vi "Tx1_Rx2_Acquisition.vi"(0 "DAQmx Device Name":tag, 1 "Tx Sampling Rate":dbl, 2 "Transmit Duration":dbl, 3 "Tx Amplitude":dbl=1.0 format="%0.2p", 5 "Tx Waveform":waveform(dbl)={"t0"=timestamp(0 s since 1904-01-01), "dt"=0.0, "Y"=[]}, 7 "AO Trigger Source":tag, 11 "error in":errorcluster, 12 "Rx Sampling Rate":dbl, 13 "Receive Duration":dbl, 14 "Voltage Rails":dbl) -> (4 "Rx Data":waveform(dbl)[](array[waveform]), 6 "Tx Waveform":waveform(dbl)(graph), 15 "error out":errorcluster)   [LabVIEW 2023]
uses:
  <vilib>/DAQmx/write.llb/DAQmx Write (Analog Wfm 1Chan NSamp).vi
  <vilib>/DAQmx/read.llb/DAQmx Read (Analog 1D Wfm NChan NSamp).vi
  <vilib>/DAQmx/create/channels.llb/DAQmx Create Channel (AO-Voltage-Basic).vi
  <vilib>/DAQmx/configure/timing.llb/DAQmx Timing (Sample Clock).vi
  <vilib>/DAQmx/configure/trigger.llb/DAQmx Start Trigger (Digital Edge).vi
  <vilib>/DAQmx/miscellaneous.llb/DAQmx Fill In Error Info.vi
  <vilib>/DAQmx/create/channels.llb/DAQmx Create Channel (AI-Voltage-Basic).vi
  <resource>/objmgr/daqmx.rc
panel:
  out "Rx Data":waveform(dbl)[](graph)
  in  "AO Channel Name":string="/ao0"
  in  "AI Channel 1 Name":string="/ai1"
  in  "AI Channel 2 Name":string="/ai2"
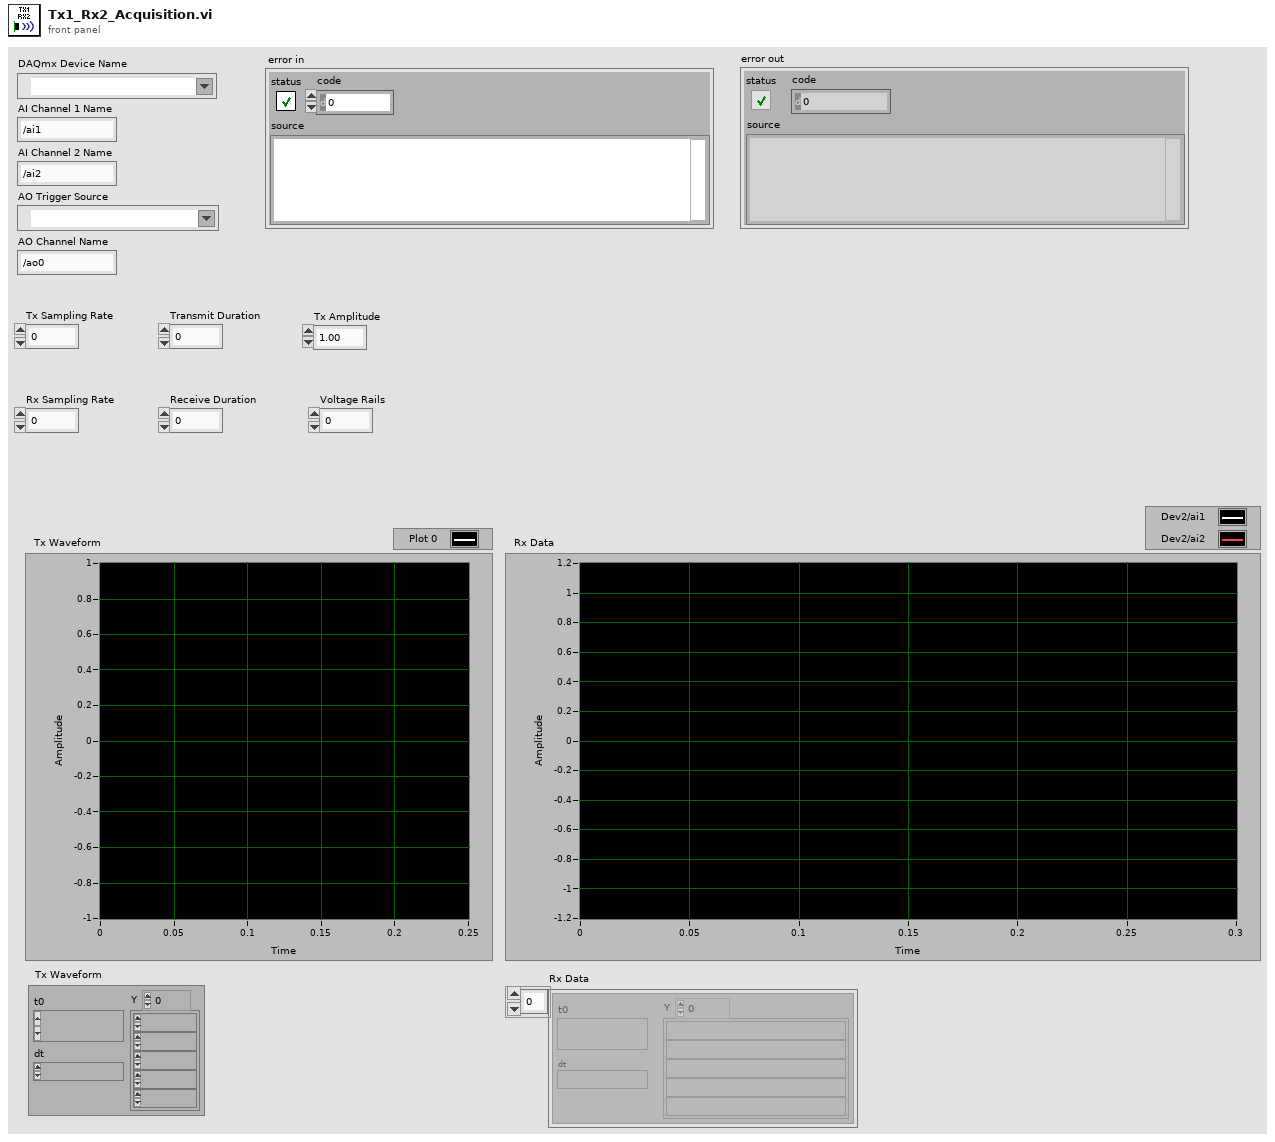
[diagram p1: front panel]
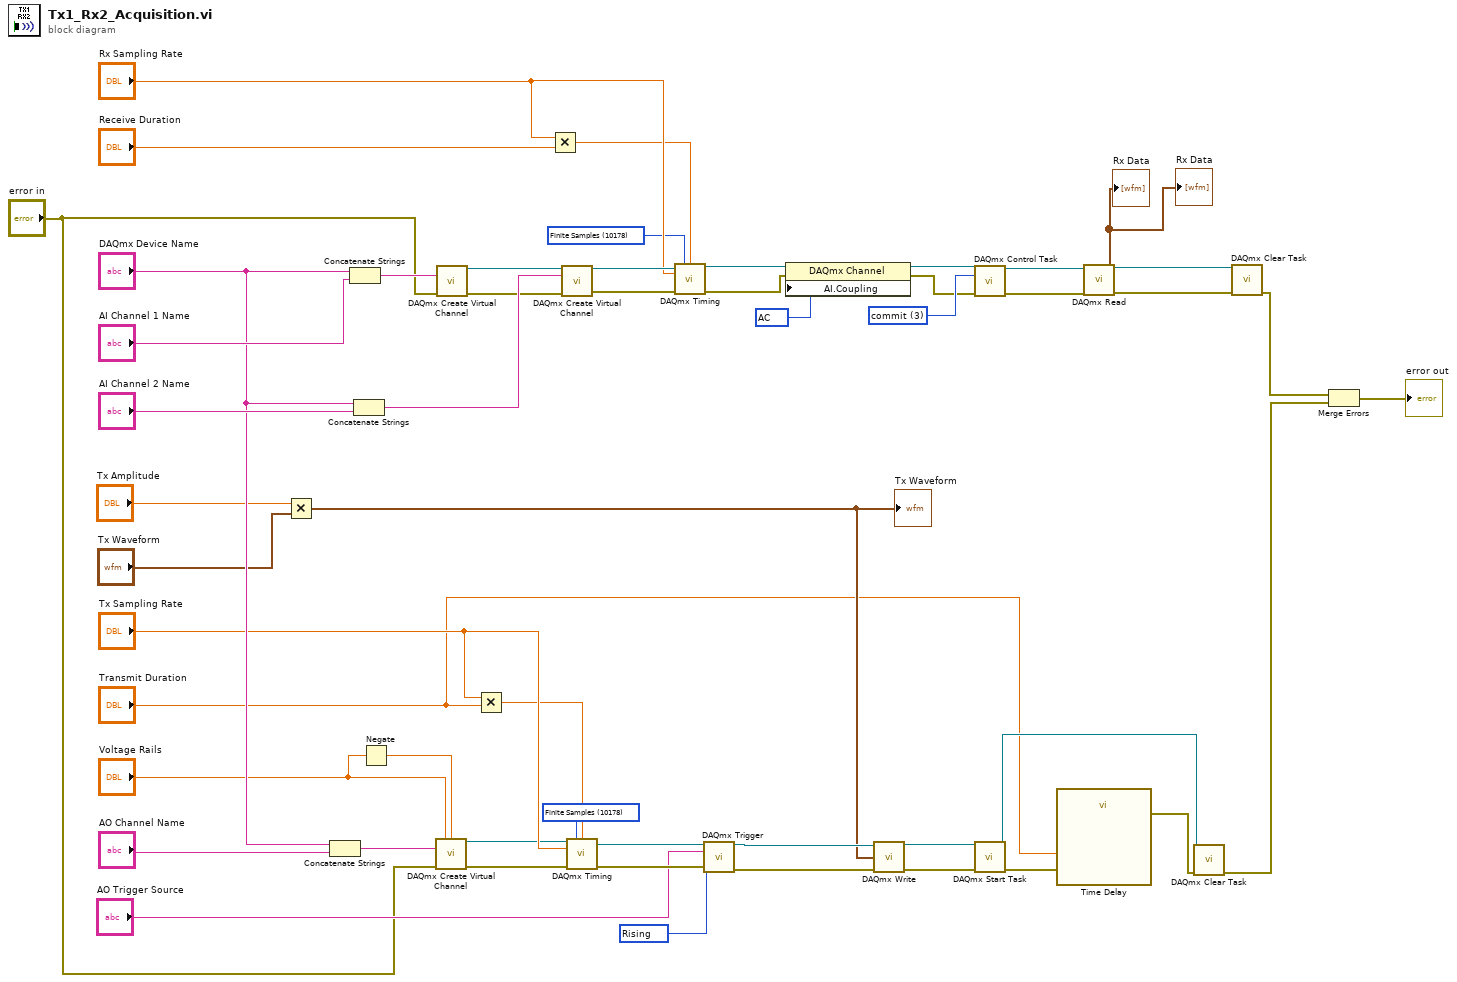
[diagram p0: block diagram]
diagram:
  w23 = 10280 items=["Rising"=10280, "Falling"=10171] ("edge")
  w25 = 10178 items=["Finite Samples"=10178, "Continuous Samples"=10123, "Hardware Timed Single Point"=12522] ("sample mode")
  w36 = 10045 items=["AC"=10045, "DC"=10050, "GND"=10066] ("AI.Coupling")
  w37 = 3 items=["verify"=2, "reserve"=4, "commit"=3, "unreserve"=5, "abort"=6] ("action")
  w40 = 10178 items=["Finite Samples"=10178, "Continuous Samples"=10123, "Hardware Timed Single Point"=12522] ("sample mode")
  n1 = Multiply(x="Tx Amplitude", y="Tx Waveform") -> (x*y=w6:waveform(dbl))
  "Tx Waveform" <- w6
  n2 = Concatenate Strings("DAQmx Device Name", "AO Channel Name") -> (w30:string)
  n3 = Concatenate Strings("DAQmx Device Name", "AI Channel 1 Name") -> (w48:string)
  n4 = Concatenate Strings("DAQmx Device Name", "AI Channel 2 Name") -> (w47:string)
  n5 = Negate(x="Voltage Rails") -> (-x=w28:dbl)
  n6 = call-poly <vilib>:"DAQmx Create Virtual Channel.vi"("maximum value"="Voltage Rails", "minimum value"=w28, "physical channels"=w30, "error in"="error in") -> ("task out"=w24:refnum<k21>, "error out"=w27:errorcluster)  [unwired: 10 in]
  n7 = call-poly <vilib>:"DAQmx Create Virtual Channel.vi"("physical channels"=w48, "error in"="error in") -> ("task out"=w46:refnum<k21>, "error out"=w45:errorcluster)  [unwired: 12 in]
  n8 = Multiply(x="Tx Sampling Rate", y="Transmit Duration") -> (x*y=w2:dbl)
  n9 = Multiply(x="Rx Sampling Rate", y="Receive Duration") -> (x*y=w41:dbl)
  n10 = call-poly <vilib>:"DAQmx Create Virtual Channel.vi"("task in"=w46, "physical channels"=w47, "error in"=w45) -> ("task out"=w44:refnum<k21>, "error out"=w32:errorcluster)  [unwired: 11 in]
  n11 = call-poly <vilib>:"DAQmx Timing.vi"("task/channels in"=w24, "sample mode"=w25, "samples per channel"=w2, "rate"="Tx Sampling Rate", "error in"=w27) -> ("task out"=w21:refnum<k21>, "error out"=w22:errorcluster)  [unwired: 9 in]
  n12 = call-poly <vilib>:"DAQmx Timing.vi"("task/channels in"=w44, "sample mode"=w40, "samples per channel"=w41, "rate"="Rx Sampling Rate", "error in"=w32) -> ("task out"=w39:refnum<k21>, "error out"=w33:errorcluster)  [unwired: 9 in]
  n13 = call-poly <vilib>:"DAQmx Trigger.vi"("task/channels in"=w21, "source"="AO Trigger Source", "edge"=w23, "error in"=w22) -> ("task out"=w19:refnum<k21>, "error out"=w18:errorcluster)  [unwired: 10 in]
  n14 = property class="DAQmx Channel"(reference=w39, error in=w33, "AI.Coupling"=w36) -> (reference out=w38:refnum<k21>, error out=w34:errorcluster)
  n15 = call-poly <vilib>:"DAQmx Write.vi"("task/channels in"=w19, "data"=w6, "error in"=w18) -> ("task out"=w15:refnum<k21>, "error out"=w14:errorcluster)  [unwired: 10 in, 1 out]
  n16 = call <vilib>:"DAQmx Control Task.vi"("task/channels in"=w38, "action"=w37, "error in"=w34) -> ("task out"=w35:refnum<k21>, "error out"=w31:errorcluster)  [unwired: 11 in]
  n17 = call <vilib>:"DAQmx Start Task.vi"("task/channels in"=w15, "error in"=w14) -> ("task out"=w9:refnum<k21>, "error out"=w4:errorcluster)  [unwired: 12 in]
  n18 = call "Time Delay"("error in (no error)"=w4, "Delay Time (s)"="Transmit Duration") -> ("error out"=w3:errorcluster)  [unwired: 9 in]
  n19 = call-poly <vilib>:"DAQmx Read.vi"("task/channels in"=w35, "error in"=w31) -> ("task out"=w13:refnum<k21>, "data"=→"Rx Data" →"Rx Data":waveform(dbl)[], "error out"=w12:errorcluster)  [unwired: 11 in]
  n20 = call <vilib>:"DAQmx Clear Task.vi"("task in"=w9, "error in"=w3) -> ("error out"=w8:errorcluster)  [unwired: 13 in]
  n21 = call <vilib>:"DAQmx Clear Task.vi"("task in"=w13, "error in"=w12) -> ("error out"=w10:errorcluster)  [unwired: 13 in]
  n22 = Merge Errors(w10, w8) -> (→"error out":errorcluster)
